vi "Calibration-Line1-CalMain.vi"(8 "error in (no error)":errorcluster, 11 "Calibration-RunTest in":refnum<class "Calibration-RunTest.lvclass">) -> (0 "error out":errorcluster, 3 "Calibration-RunTest out":refnum<class "Calibration-RunTest.lvclass">)   [LabVIEW 2013, in "Calibration-RunTest.lvclass"]
uses:
  Calibration-RunTest.lvclass
  Calibration-RunTest.lvclass/Calibration-RunTest.ctl
  Motion Control/Motion-ControlAll.lvclass
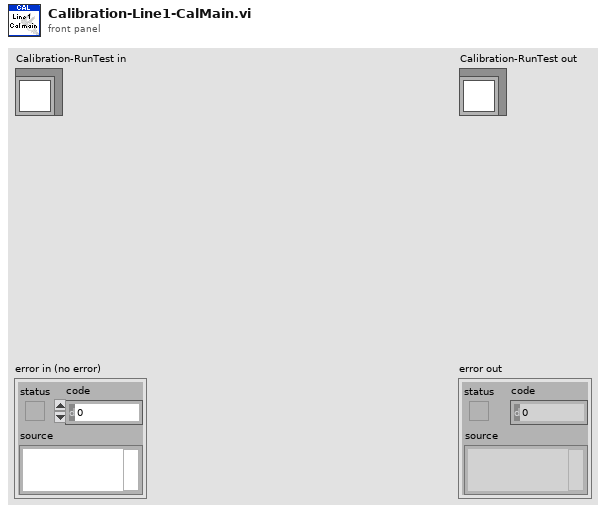
[diagram p1: front panel]
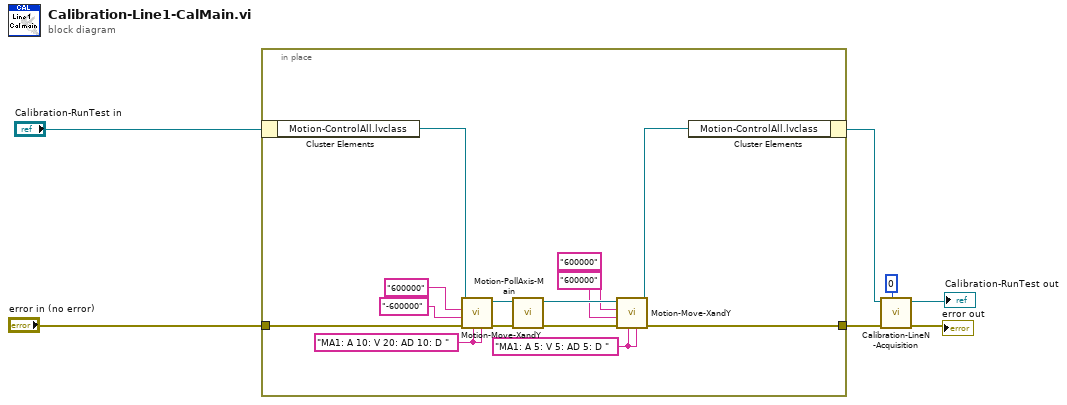
[diagram p0: block diagram]
diagram:
  n1 = in-place {
    in-place-border: "error in (no error)" -> [w10]
    in-place-border: [w8] -> w4
    w21 = "MA1: A 10: V 20: AD 10: D " ("concatenated string")
    w20 = "MA1: A 5: V 5: AD 5: D " ("concatenated string")
    n2 = in-place-cluster #1("Calibration-RunTest in") -> ("Motion-ControlAll.lvclass"=w11:refnum<class "Motion-ControlAll.lvclass">)
    n3 = call "Motion-Move-XandY.vi"("Y Drive Acc/Speed/Velocity"=w21, "X Drive Acc/Speed/Velocity"=w21, "error in (no error)"=w10, "X Coordinates"="-600000", "Y Coordinates"="600000", "Motion-ControlAll in"=w11) -> ("error out"=w13:errorcluster, "Motion-ControlAll out"=w12:refnum<class "Motion-ControlAll.lvclass">)  [unwired: 4 in]
    n4 = call "Motion-PollAxis-Main.vi"("error in (no error)"=w13, "Motion-ControlAll in"=w12) -> ("error out"=w18:errorcluster, "Motion-ControlAll out"=w19:refnum<class "Motion-ControlAll.lvclass">)  [unwired: 8 in]
    n5 = call "Motion-Move-XandY.vi"("Y Drive Acc/Speed/Velocity"=w20, "X Drive Acc/Speed/Velocity"=w20, "error in (no error)"=w18, "X Coordinates"="600000", "Y Coordinates"="600000", "Motion-ControlAll in"=w19) -> ("error out"=w8:errorcluster, "Motion-ControlAll out"=w9:refnum<class "Motion-ControlAll.lvclass">)  [unwired: 4 in]
    n6 = in-place-cluster #1("Motion-ControlAll.lvclass"=w9) -> (w3:refnum<class "Calibration-RunTest.lvclass">)
  }
  n7 = call "Calibration-LineN-Acquisition.vi"("Cal Line?"=0, "error in (no error)"=w4, "Calibration-RunTest in"=w3) -> ("error out"=→"error out":errorcluster, "Calibration-RunTest out"=→"Calibration-RunTest out":refnum<class "Calibration-RunTest.lvclass">)  [unwired: 7 in]
